vi "Resize.vi"(10 "Number of Rows (auto from ref)":i32=-1, 11 "Cyclic Table in":refnum<class "Cyclic Table.lvclass">) -> (3 "Cyclic Table out":refnum<class "Cyclic Table.lvclass">)   [LabVIEW 2024, in "Cyclic Table.lvclass"]
doc: "Trigger a resize of the Cyclic Table buffer, matching the number of visible rows in the Table Control provided in \"Initialize.vi\". This VI should be called to handle resizing events of the Table Control (such as \"Pane\": Pane Size if the Table Control resizes with the pane)."
uses:
  Cyclic Table.lvclass
  Cyclic Table.lvclass/Cyclic Table.ctl
  Update Method.ctl
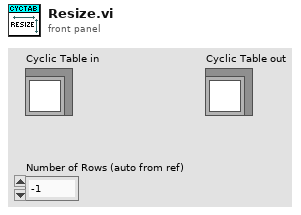
[diagram p1: front panel]
types:
  T1 = typedef "Cyclic Table.lvclass/Update Method.ctl" = enum16{"Cyclic", "Old Top", "New Top"}
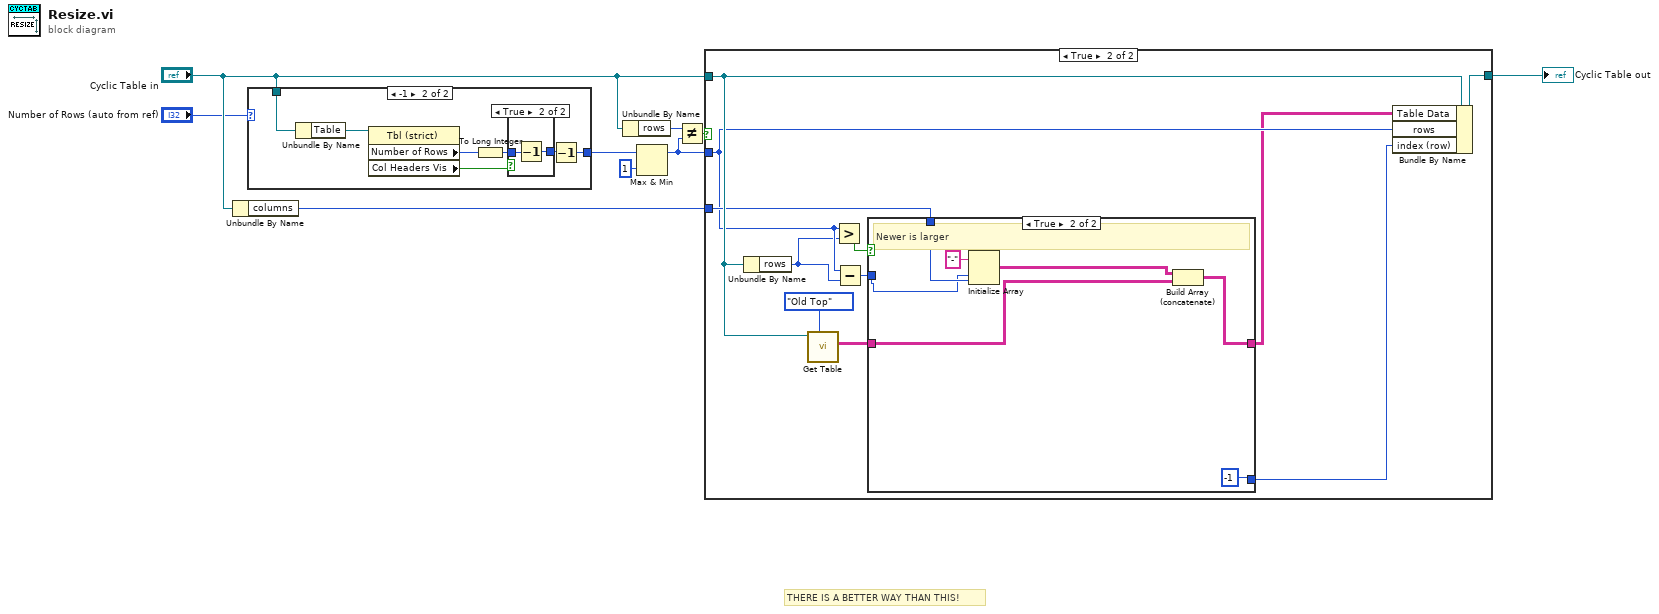
[diagram p0: block diagram]
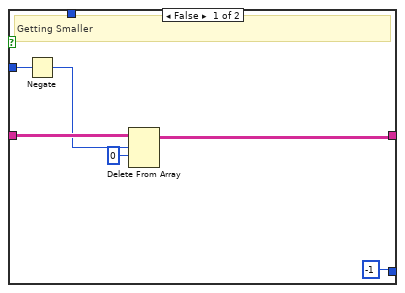
[diagram p5: hidden frame]
diagram:
  # "THERE IS A BETTER WAY THAN THIS!"
  n1 = Unbundle By Name("Cyclic Table in") -> ("columns"=w5:i32)
  n2 = case shown="-1" "Number of Rows (auto from ref)" {
    selector: "Number of Rows (auto from ref)" -> [w10 _]
    tunnel: "Cyclic Table in" -> [_ w12]
    tunnel: [w10 w11] -> w1
    frame Default {
    }
    frame -1 {
      n3 = Unbundle By Name(w12) -> ("Table"=w16:refnum<vi>)
      n4 = property on="Property Node" class="Tbl (strict)"(reference=w16) -> ("Number of Rows"=w17:u32, "Col Headers Vis"=w13:bool)  [unwired: 1 in, 2 out]
      n5 = To Long Integer(number=w17) -> (32bit integer=w15:i32)
      n6 = case shown="True" w13 {
        tunnel: w15 -> [w18 w20]
        tunnel: [w18 w19] -> w14
        frame False {
        }
        frame True {
          n7 = Decrement(x=w20) -> (x-1=w19:i32)
        }
      }
      n8 = Decrement(x=w14) -> (x-1=w11:i32)
    }
  }
  n9 = Unbundle By Name("Cyclic Table in") -> ("rows"=w4:i32)
  n10 = Max & Min(x=w1, y=1 ("lower limit")) -> (max(x,y)=w3:i32)  [unwired: 1 out]
  n11 = Not Equal?(x=w4, y=w3) -> (x != y?=w2:bool)
  n12 = case shown="True" w2 {
    tunnel: [w21 w32] -> w8
    tunnel: w5 -> [_ w27]
    tunnel: "Cyclic Table in" -> [w21 w29]
    tunnel: w3 -> [_ w26]
    frame False {
    }
    frame True {
      n13 = Unbundle By Name(w29) -> ("rows"=w23:i32)
      n14 = call "Get Table.vi"("Update Method (New Top)"=Update_Method."Old Top", "Cyclic Table in"=w29) -> ("Table Data (sorted by time)"=w24:string[][])  [unwired: 9 in]
      n15 = Greater?(x=w26, y=w23) -> (0:w31:bool)
      n16 = Subtract(x=w26, y=w23) -> (x-y=w22:i32)
      n17 = case shown="True" w31 {
        tunnel: [-1 ("index (row)") -1 ("index (row)")] -> w30
        tunnel: w24 -> [w36 w41]
        tunnel: [w37 w40] -> w25
        tunnel: w27 -> [_ w43]
        tunnel: w22 -> [w35 w39]
        frame False {
          # "Getting Smaller"
          n18 = Negate(x=w35) -> (-x=w34:i32)
          n19 = Delete From Array(array=w36, length=w34, index (row)=0) -> (array with subset deleted=w37:string[][])  [unwired: 1 in, 1 out]
        }
        frame True {
          # "Newer is larger"
          n20 = Initialize Array("-" ("Message Class"), w39, w43) -> (w42:string[][])
          n21 = Build Array (concatenate)(w42, w41) -> (w40:string[][])
        }
      }
      n22 = Bundle By Name(cluster=w29, "Table Data"=w25, "rows"=w26, "index (row)"=w30) -> (w32:refnum<class "Cyclic Table.lvclass">)
    }
  }
  "Cyclic Table out" <- w8
